vi "Constructor.vi"(8 "error in (no error)":errorcluster, 11 "FAMM in":refnum<class "FAMM.lvclass">) -> (0 "error out":errorcluster, 3 "FAMM out":refnum<class "FAMM.lvclass">)   [LabVIEW 2014, in "FAMM.lvclass"]
uses:
  FAMM.lvclass
  DBAL/DBAL.lvclass
  FAMM.lvclass/FAMM.ctl
  PAQ-memory.lvclass
  AVPP/AVPP.lvclass
  HISW/HISW.lvclass
  Common/controls/GlobalClassRefs.vi
panel:
  out "PAQ layers":i32
  out "PAQ rate":dbl
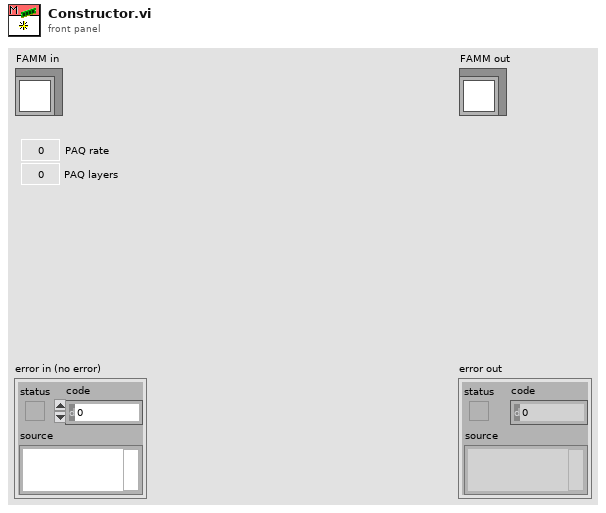
[diagram p1: front panel]
types:
  T1 = cluster{"Time":refnum<data-value>, "TAGdata":cluster{"source":refnum<data-value>, "status":refnum<data-value>, "data":refnum<data-value>, "max":refnum<data-value>, "min":refnum<data-value>}[]}
  T2 = cluster{"Size":i32, "Layer":i32, "TableName":string}
  T3 = cluster{"source":refnum<data-value>, "status":refnum<data-value>, "data":refnum<data-value>, "max":refnum<data-value>, "min":refnum<data-value>}[]
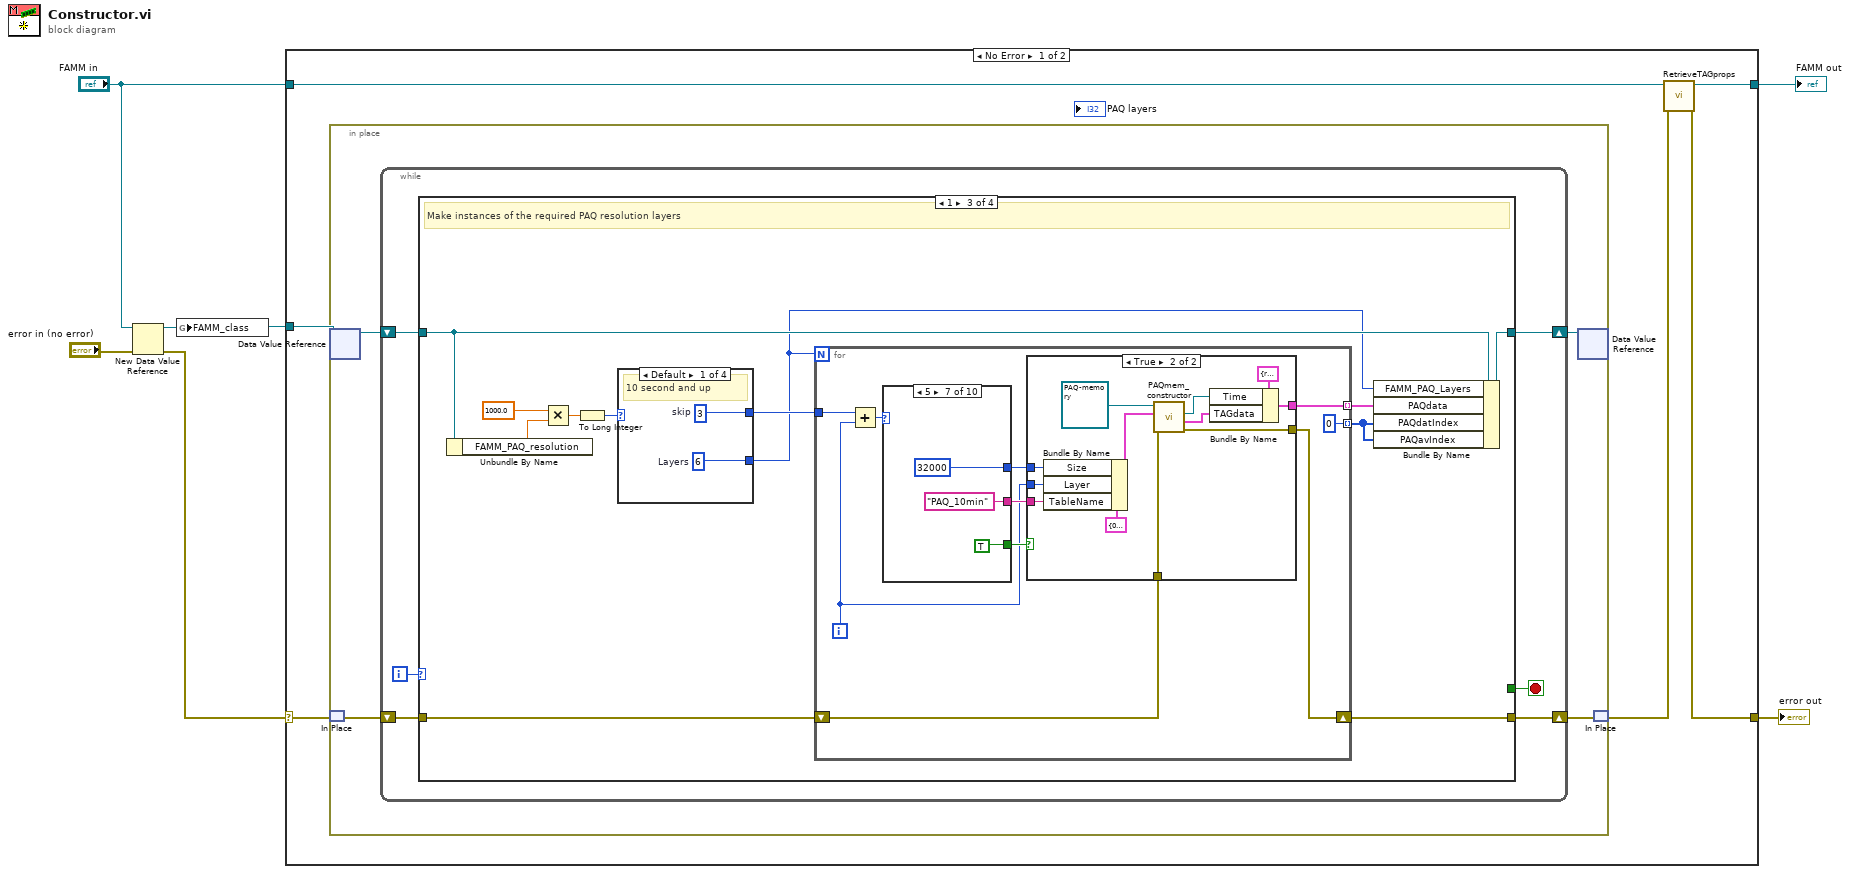
[diagram p0: block diagram]
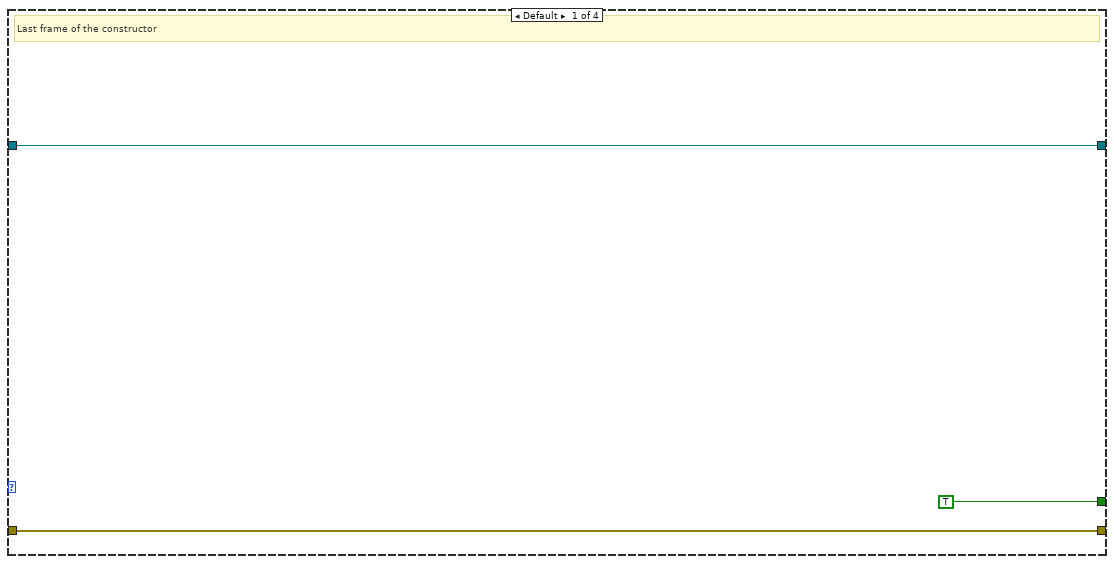
[diagram p2: hidden frame]
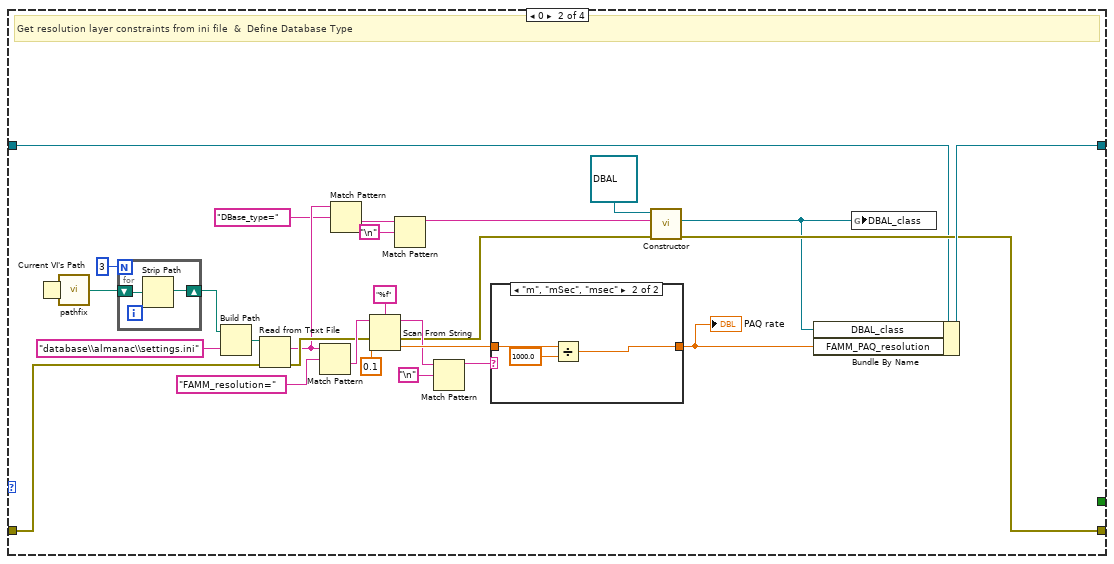
[diagram p3: hidden frame]
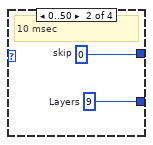
[diagram p5: hidden frame]
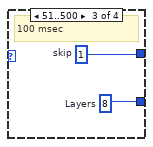
[diagram p6: hidden frame]
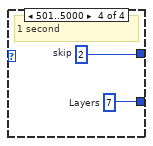
[diagram p7: hidden frame]
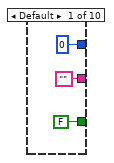
[diagram p9: hidden frame]
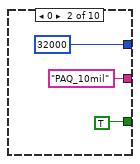
[diagram p10: hidden frame]
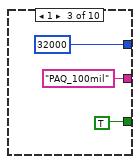
[diagram p11: hidden frame]
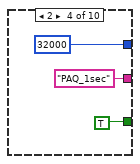
[diagram p12: hidden frame]
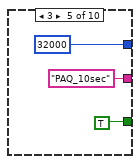
[diagram p13: hidden frame]
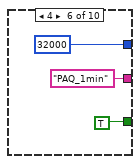
[diagram p14: hidden frame]
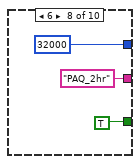
[diagram p15: hidden frame]
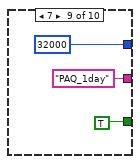
[diagram p16: hidden frame]
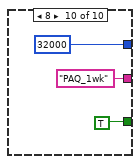
[diagram p17: hidden frame]
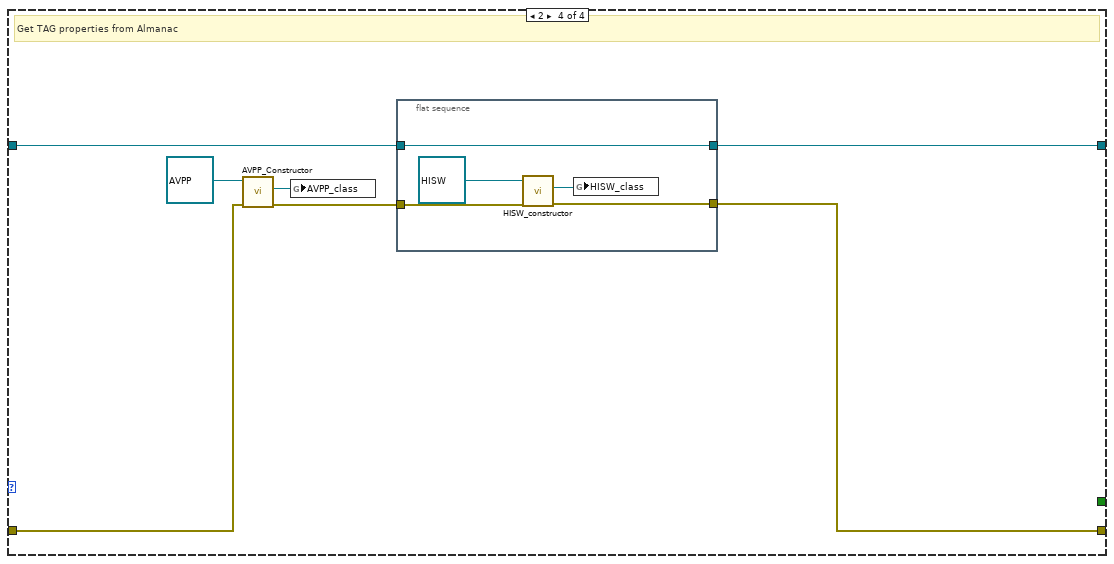
[diagram p18: hidden frame]
diagram:
  n1 = New Data Value Reference(data value="FAMM in", error in="error in (no error)") -> (data value reference=w1:refnum<data-value>, error out=w3:errorcluster)
  n2 = global write "GlobalClassRefs.vi" "FAMM_class"(w1) -> ()
  n3 = case shown="No Error" w3 {
    selector: w3 -> [w11 w145]
    tunnel: [w7 w145] -> w6
    tunnel: "FAMM in" -> [w10 w144]
    tunnel: [w9 w144] -> w2
    tunnel: w1 -> [w12 _]
    frame No Error {
      n4 = in-place {
        n5 = in-place-dvr #1(w12) -> (w16:refnum<class "FAMM.lvclass">)  [unwired: 1 out]
        n6 = in-place-match #2(w11) -> (w15:errorcluster)
        n7 = while {
          shift-right: [w20] -> w14
          shift-left: w16 -> [w21]
          shift-right: [w18] -> w13
          shift-left: w15 -> [w19]
          i -> [w22]
          stop <- w17 stop-if-true
          n8 = case shown="1" w22 {
            tunnel: w21 -> [w25 w28 w63 w134]
            tunnel: [w25 w39 w62 w133] -> w20
            tunnel: w19 -> [w24 w27 w66 w137]
            tunnel: [w24 w30 w65 w132] -> w18
            tunnel: [TRUE _ _ _] -> w17
            frame Default {
              # "Last frame of the constructor"
            }
            frame 0 {
              # "Get resolution layer constraints from ini file  &  Define Database Type"
              n9 = Current VI's Path() -> (path=w53:path)
              n10 = call "pathfix.vi"("Current VI's Path"=w53) -> ("Fixed path"=w52:path)  [unwired: 4 in]
              n11 = for {
                N: 3 -> [_]
                shift-right: [w58] -> w50
                shift-left: w52 -> [w59]
                n12 = Strip Path(path=w59) -> (stripped path=w58:path)  [unwired: 1 out]
              }
              n13 = Build Path(base path=w50, name or relative path="database\\almanac\\settings.ini") -> (appended path=w48:path)
              n14 = Read from Text File(file (use dialog)=w48, error in=w27) -> (text=w35:string, error out=w38:errorcluster)  [unwired: 2 in, 2 out]
              n15 = Match Pattern(string=w35, regular expression="FAMM_resolution=" ("format string")) -> (after substring=w45:string)  [unwired: 1 in, 3 out]
              n16 = Match Pattern(string=w35, regular expression="DBase_type=" ("format string")) -> (after substring=w32:string)  [unwired: 1 in, 3 out]
              n17 = Scan From String(format string="%f", input string=w45, error in=w38, default 1=0.1 ("default value 1")) -> (remaining string=w41:string, error out=w26:errorcluster, output 1=w43:dbl)  [unwired: 1 in, 1 out]
              n18 = Match Pattern(string=w32, regular expression="\n") -> (before substring=w31:string)  [unwired: 1 in, 3 out]
              n19 = Match Pattern(string=w41, regular expression="\n") -> (before substring=w42:string)  [unwired: 1 in, 3 out]
              n20 = case shown="\"m\", \"mSec\", \"msec\"" w42 {
                tunnel: w43 -> [w54 w57]
                tunnel: [w54 w55] -> w40
                frame Default {
                }
                frame "m", "mSec", "msec" {
                  n21 = Divide(x=w57, y=1000.0) -> (x/y=w55:dbl)
                }
              }
              "PAQ rate" <- w40
              n22 = call "Constructor.vi"("error in (no error)"=w26, "DatabaseType"=w31, "DBAL in"=refnum<class "DBAL.lvclass"> refnum) -> ("error out"=w30:errorcluster, "DBAL_class"=w29:refnum<data-value>)  [unwired: 6 in, 1 out]
              n23 = Bundle By Name(cluster=w28, "DBAL_class"=w29, "FAMM_PAQ_resolution"=w40) -> (w39:refnum<class "FAMM.lvclass">)
              n24 = global write "GlobalClassRefs.vi" "DBAL_class"(w29) -> ()
            }
            frame 1 {
              # "Make instances of the required PAQ resolution layers"
              n25 = Unbundle By Name(w63) -> ("FAMM_PAQ_resolution"=w71:dbl)
              n26 = Multiply(x=1000.0, y=w71) -> (x*y=w69:dbl)
              n27 = To Long Integer(number=w69) -> (32bit integer=w68:i32)
              n28 = case shown="Default" w68 {
                tunnel: [w73 w75 w77 w79] -> w67
                tunnel: [w72 w74 w76 w78] -> w60
                frame Default {
                  w72 = 6  # Layers
                  w73 = 3  # skip
                  # "10 second and up"
                }
                frame 0..50 {
                  w74 = 9  # Layers
                  w75 = 0  # skip
                  # "10 msec"
                }
                frame 51..500 {
                  w76 = 8  # Layers
                  w77 = 1  # skip
                  # "100 msec"
                }
                frame 501..5000 {
                  w78 = 7  # Layers
                  w79 = 2  # skip
                  # "1 second"
                }
              }
              n29 = for {
                N: w60 -> [_]
                tunnel: w67 -> [w89]
                shift-right: [w82] -> w65
                shift-left: w66 -> [w88]
                tunnel: [w81] -> w64 mode=indexing
                tunnel: [0 ("Pointer")] -> w61 mode=indexing
                i -> [w83]
                n30 = Add(x=w89, y=w83) -> (x+y=w87:i32)
                n31 = case shown="5" w87 {
                  tunnel: [0 ("Size") 32000 ("Size") 32000 ("Size") 32000 ("Size") 32000 ("Size") 32000 ("Size") 32000 ("Size") 32000 ("Size") 32000 ("Size") 32000 ("Size")] -> w86
                  tunnel: [FALSE TRUE TRUE TRUE TRUE TRUE TRUE TRUE TRUE TRUE] -> w85
                  tunnel: ["" "PAQ_10mil" "PAQ_100mil" "PAQ_1sec" "PAQ_10sec" "PAQ_1min" "PAQ_10min" "PAQ_2hr" "PAQ_1day" "PAQ_1wk"] -> w84
                  frame Default {
                  }
                  frame 0 {
                  }
                  frame 1 {
                  }
                  frame 2 {
                  }
                  frame 3 {
                  }
                  frame 4 {
                  }
                  frame 5 {
                  }
                  frame 6 {
                  }
                  frame 7 {
                  }
                  frame 8 {
                  }
                }
                n32 = case shown="True" w85 {
                  tunnel: w88 -> [_ w98]
                  tunnel: w86 -> [_ w97]
                  tunnel: w83 -> [_ w96]
                  tunnel: w84 -> [_ w95]
                  tunnel: [_ w94] -> w82
                  tunnel: [_ w90] -> w81
                  frame False {
                  }
                  frame True {
                    n33 = Bundle By Name(cluster=T2 {"Size"=0, "Layer"=0, "TableName"=""} ("LayerInfo"), "Size"=w97, "Layer"=w96, "TableName"=w95) -> (w99:T2)
                    n34 = call-dynamic "PAQmem_constructor.vi"("error in (no error)"=w98, "LayerInfo"=w99, "PAQ-memory in"=refnum<class "PAQ-memory.lvclass"> refnum) -> ("error out"=w94:errorcluster, "TAGdata"=w92:T3, "Time"=w91:refnum<data-value>)  [unwired: 5 in, 1 out]
                    n35 = Bundle By Name(cluster=T1 {"Time"=refnum, "TAGdata"=[]} ("PAQlayer"), "Time"=w91, "TAGdata"=w92) -> (w90:T1)
                  }
                }
              }
              n36 = Bundle By Name(cluster=w63, "FAMM_PAQ_Layers"=w60, "PAQdata"=w64, "PAQdatIndex"=w61, "PAQavIndex"=w61) -> (w62:refnum<class "FAMM.lvclass">)
            }
            frame 2 {
              # "Get TAG properties from Almanac"
              n37 = call "AVPP_Constructor.vi"("error in (no error)"=w137, "AVPP in"=refnum<class "AVPP.lvclass"> refnum) -> ("error out"=w135:errorcluster, "AVPP_ref"=w136:refnum<data-value>)  [unwired: 7 in, 1 out]
              n38 = global write "GlobalClassRefs.vi" "AVPP_class"(w136) -> ()
              n39 = flat-sequence {
                tunnel: w135 -> [w142]
                tunnel: [w141] -> w132
                tunnel: w134 -> [w140]
                tunnel: [w140] -> w133
                frame #0 {
                  n40 = call "HISW_constructor.vi"("error in (no error)"=w142, "HISW in"=refnum<class "HISW.lvclass"> refnum) -> ("error out"=w141:errorcluster, "HISW_ref"=w139:refnum<data-value>)  [unwired: 7 in, 1 out]
                  n41 = global write "GlobalClassRefs.vi" "HISW_class"(w139) -> ()
                }
              }
            }
          }
        }
        n42 = in-place-dvr #1(w14) -> ()  [unwired: 2 out]
        n43 = in-place-match #2(w13) -> (w8:errorcluster)
      }
      n44 = call "RetrieveTAGprops.vi"("error in (no error)"=w8, "FAMM in"=w10) -> ("error out"=w7:errorcluster, "FAMM out"=w9:refnum<class "FAMM.lvclass">)  [unwired: 8 in]
    }
    frame Error {
    }
  }
  "error out" <- w6
  "FAMM out" <- w2
